vi "CRYCheck Freq Option.vi"(9 "Option Array In":bool[](array[boolean]), 10 "Averaging":u16, 11 "Algorithm":u16) -> (3 "Option Array Out":bool[](array[boolean]))   [LabVIEW 2013]
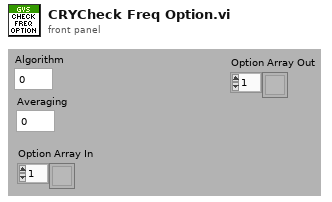
[diagram p1: front panel]
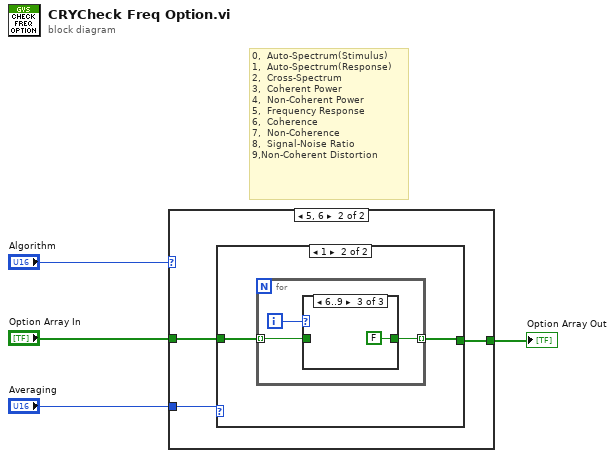
[diagram p0: block diagram]
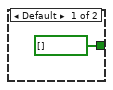
[diagram p2: hidden frame]
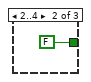
[diagram p5: hidden frame]
diagram:
  # "0,  Auto-Spectrum(Stimulus)\n1,  Auto-Spectrum(Response)\n2,  Cross-Spectrum\n3,  Coherent Power\n4,  Non-Coherent Power\n5,  Frequency Response\n6,  Coherence\n7,  Non-Coherence\n8,  Signal-Noise Ratio\n9,Non-Coherent Distortion"
  n1 = case shown="5, 6" "Algorithm" {
    tunnel: "Option Array In" -> [_ w8]
    tunnel: "Averaging" -> [_ w7]
    tunnel: [bool[] [] w6] -> w1
    frame Default {
    }
    frame 5, 6 {
      n2 = case shown="1" w7 {
        tunnel: w8 -> [w9 w11]
        tunnel: [w9 w10] -> w6
        frame 0, Default {
        }
        frame 1 {
          n3 = for {
            tunnel: w11 -> [w13] mode=indexing
            tunnel: [w12] -> w10 mode=indexing
            i -> [w14]
            n4 = case shown="6..9" w14 {
              tunnel: w13 -> [w15 _ _]
              tunnel: [w15 FALSE ("Is Har meas.freq? 2") FALSE ("Is Har meas.freq? 2")] -> w12
              frame Default {
              }
              frame 2..4 {
              }
              frame 6..9 {
              }
            }
          }
        }
      }
    }
  }
  "Option Array Out" <- w1
